vi "Get Comment.vi"(8 "error in (no error)":errorcluster, 11 "PropertyObject in":refnum<class "PropertyObject.lvclass">) -> (0 "error out":errorcluster, 2 "Comment":string, 3 "PropertyObject out":refnum<class "PropertyObject.lvclass">)   [LabVIEW 2020, in "TSnax.lvlib" / "PropertyObject.lvclass"]
uses:
  PropertyObject.lvclass
  PropertyObject.lvclass/PropertyObject.ctl
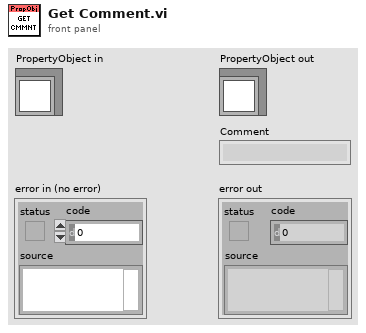
[diagram p1: front panel]
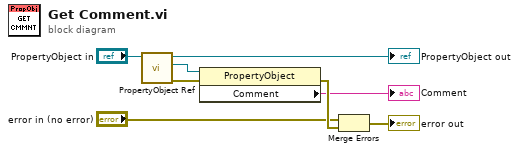
[diagram p0: block diagram]
diagram:
  n1 = call "PropertyObject Ref.vi"("PropertyObject in"="PropertyObject in") -> ("error out"=w7:errorcluster, "PropertyObject"=w8:refnum<k7>, "PropertyObject out"=→"PropertyObject out":refnum<class "PropertyObject.lvclass">)  [unwired: 8 in]
  n2 = property class="PropertyObject"(reference=w8, error in=w7) -> (error out=w6:errorcluster, "Comment"=→"Comment":string)  [unwired: 1 out]
  n3 = Merge Errors("error in (no error)", w6) -> (→"error out":errorcluster)
